vi "PicoScopeospaRunBlock.vi"(7 "Acquisition Settings":T1={"preTriggerSamples"=0, "postTriggerSamples"=1000, "timebase"=2} {"postTriggerSamples" format="%_6p"; "preTriggerSamples" format="%_6p"}, 8 "error in (no error)":errorcluster, 11 "handle in":i16) -> (0 "error out":errorcluster, 3 "handle out":i16, 4 "timeIndisposedMs":dbl, 6 "Total Requested Samples":u64)   [LabVIEW 2010]
doc: "Calls RunBlock"
uses:
  psospa.dll
  shared/Acquisition Settings.ctl
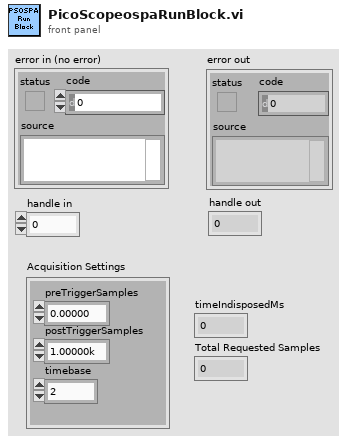
[diagram p1: front panel]
types:
  T1 = typedef "Acquisition Settings.ctl" = cluster{"preTriggerSamples":u64, "postTriggerSamples":u64, "timebase":u32}
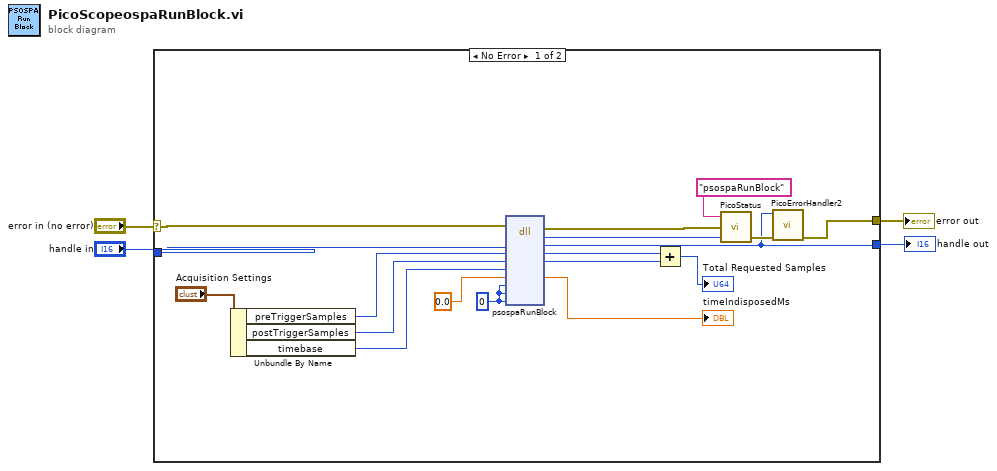
[diagram p0: block diagram]
diagram:
  n1 = case shown="No Error" "error in (no error)" {
    selector: "error in (no error)" -> [w16 w24]
    tunnel: [w10 w24] -> w2
    tunnel: "handle in" -> [w15 w23]
    tunnel: [w9 w23] -> w3
    frame No Error {
      w5 = u64 0 ("pParameter")
      n2 = Unbundle By Name("Acquisition Settings") -> ("preTriggerSamples"=w14:u64, "postTriggerSamples"=w13:u64, "timebase"=w12:u32)
      n3 = dll-call lib="psospa.dll" fn="psospaRunBlock" ("ps3000.dll:_ps3000_open_unit@0")(error in=w16, "handle"=w15, "noOfPreTriggerSamples"=w14, "noOfPostTriggerSamples"=w13, "timebase"=w12, "timeIndisposedMs"=0.0 ("pParameter"), "segmentIndex"=w5, "lpReady"=w5, "pParameter"=w5) -> (error out=w18:errorcluster, "PICO_STATUS"=w19:u32, "handle"=w9:i16, "noOfPreTriggerSamples"=w22:u64, "noOfPostTriggerSamples"=w21:u64, "timeIndisposedMs"=→"timeIndisposedMs":dbl)  [unwired: 6 in, 1 out]
      n4 = Add(x=w22, y=w21) -> (x+y=→"Total Requested Samples":u64)
      n5 = call "PicoStatus.vi"("PICO STATUS"=w19, "error in"=w18, "source"="psospaRunBlock") -> ("error out"=w11:errorcluster)
      n6 = call "PicoErrorHandler2.vi"("error in (no error)"=w11, "handle In"=w9) -> ("error out"=w10:errorcluster)  [unwired: 9 in]
    }
    frame Error {
    }
  }
  "error out" <- w2
  "handle out" <- w3
